vi "Drive Train Global.vi"() -> ()   [LabVIEW 2018]
panel:
  in  "Robot Slow Threshold":dbl=25.0
  in  "Robot Slow?":bool=TRUE
  in  "Robot Stopped?":bool=TRUE
  in  "Reset Field Position":bool
  in  "Wheel Angle Offsets Practice Bot":T1={"FrontLeft"=-114.2, "FrontRight"=-153.9, "BackLeft"=-23.0, "BackRight"=-19.1}
  in  "Angle Locking to":dbl=540.0
  in  "Angle to Lock To":dbl=180.0
  out "Lock to Angle":bool
  out "Robot Centric":bool
  in  "Don't Turn While Translate PID Gains":T2 {"derivative time (Td, min)" format="%.3f"; "integral time (Ti, min)" format="%.3f"; "proportional gain (Kc)" format="%.3f"}
  in  "Zero Yaw":bool
  in  "Wheel Angle Offsets":T1={"FrontLeft"=135.2, "FrontRight"=36.9, "BackLeft"=116.6, "BackRight"=138.8}
  out "Wheel Angles":T1={"FrontLeft"=272.99541364540335, "FrontRight"=-87.7839585043923, "BackLeft"=273.2398027297803, "BackRight"=267.46375482727285}
  in  "Rot. Point Y":dbl
  in  "Rot. Point X":dbl
  in  "Wheel Turn PID Values":T3={"Front Left"={"P Value"=0.014, "I Value"=0.0, "D Value"=0.0}, "Front Right"={"P Value"=0.014, "I Value"=0.0, "D Value"=0.0}, "Back Left"={"P Value"=0.014, "I Value"=0.0, "D Value"=0.0}, "Back Right"={"P Value"=0.014, "I Value"=0.0, "D Value"=0.0}}
  in  "Z Command":dbl=-0.07874015748031496
  in  "Y Command":dbl=-0.0
  out "Gyro Information":T4={"Rollover"=0.0, "Yaw"=-4.26, "Cont Yaw"=-4.26}
  in  "X Command":dbl
  in  "Current State":enum16{"Reached Position", "Going to Position"}(ring)
  in  "Current Mode":T5(ring)=enum."Field Oriented"
  out "Extra Info":bool
  out "Velocity":cluster{"X":dbl, "Y":dbl}
  out "Position":cluster{"X":dbl, "Y":dbl}={"X"=0.0004896522252429492, "Y"=6.565293738080478e-06}
  out "Wheel Drive Encoders":cluster{"Rates":dbl[], "Distances":dbl[]}={"Rates"=[0.0, 0.0, -0.0, -0.0], "Distances"=[195.26625, 229.86928250000003, -80.247456, 179.07341]}
  # "X Command is spin"
  # "Z is X"
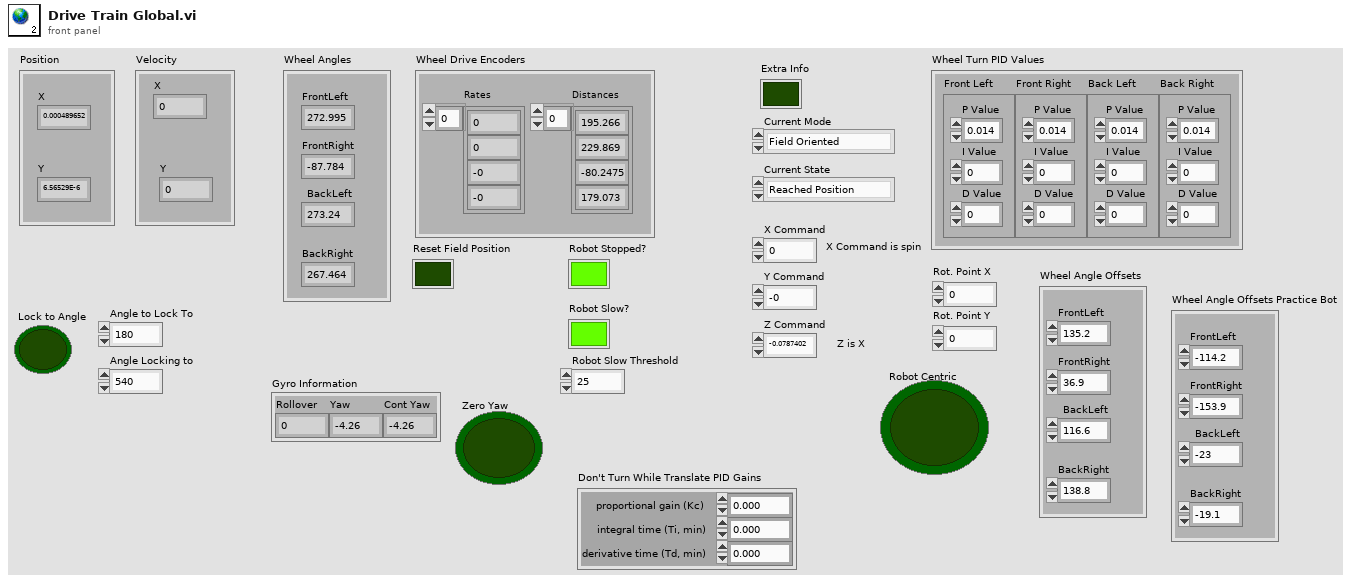
[diagram p1: front panel]
types:
  T1 = cluster{"FrontLeft":dbl, "FrontRight":dbl, "BackLeft":dbl, "BackRight":dbl}
  T2 = cluster{"proportional gain (Kc)":dbl, "integral time (Ti, min)":dbl, "derivative time (Td, min)":dbl}
  T3 = cluster{"Front Left":cluster{"P Value":dbl, "I Value":dbl, "D Value":dbl}, "Front Right":cluster{"P Value":dbl, "I Value":dbl, "D Value":dbl}, "Back Left":cluster{"P Value":dbl, "I Value":dbl, "D Value":dbl}, "Back Right":cluster{"P Value":dbl, "I Value":dbl, "D Value":dbl}}
  T4 = cluster{"Rollover":dbl, "Yaw":dbl, "Cont Yaw":dbl}
  T5 = enum16{"Autonomous Mode", "Field Oriented", "Robot Oriented", "Tank Mode"}
diagram:
